vi "Write_SIDto_global_ini.vi"(8 "Error In":errorcluster, 9 "Session id name":string="sid", 10 "SID":string, 11 "Global ini path":path) -> (0 "Error Out":errorcluster)   [LabVIEW 2017]
doc: "This VI records the SID at runtime and place it in Global ini file\n\n\\..\\UltraSonic_Test_Scripts\\UltraSonic_Global_Config.ini"
uses:
  <vilib>/Utility/config.llb/Write Key (String).vi
  <vilib>/Utility/config.llb/NI_LVConfig.lvlib
panel:
  out "found?":bool
  # "WRITE SID TO GLOBAL INI FILE"
  # "ERROR"
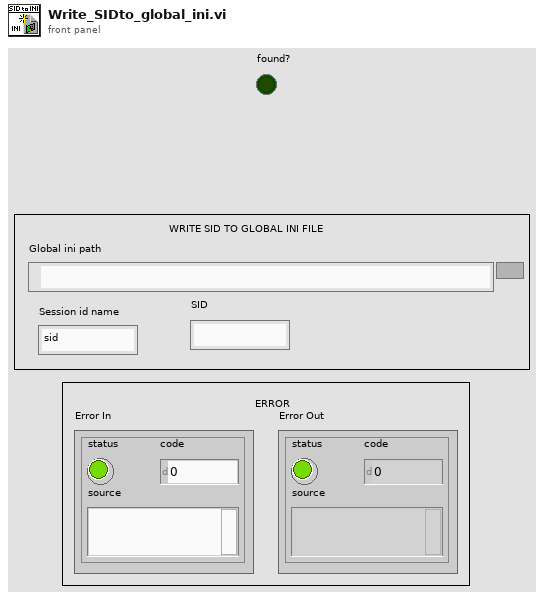
[diagram p1: front panel]
types:
  T1 = typedef "NI_LVConfig.lvlib/Config Data RefNum.ctl" = refnum<k1>
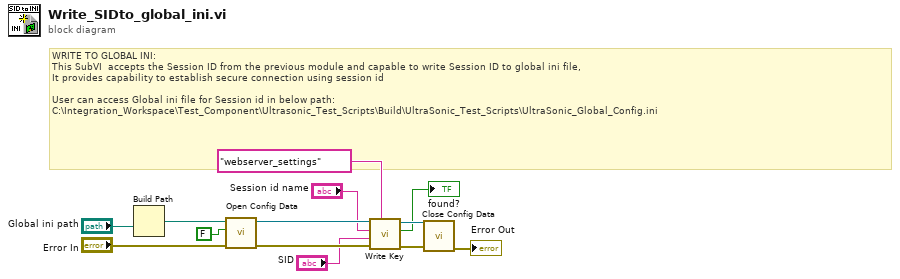
[diagram p0: block diagram]
diagram:
  # "WRITE TO GLOBAL INI:\nThis SubVI  accepts the Session ID from the previous module and capable to write Session ID to global ini file, \nIt provides capability to establish secure connection using session id\n\nUser can access Global ini file for Session id in below path:\nC:\\Integration_Workspace\\Test_Component\\Ultrasonic_Test_Scripts\\Build\\UltraSonic_Test_Scripts\\UltraSonic_Global_Config.ini"
  n1 = Build Path(name or relative path="Global ini path") -> (appended path=w12:path)  [unwired: 1 in]
  n2 = call <vilib>:"Open Config Data.vi"("error in (no error)"="Error In", "create file if necessary (T)"=FALSE ("create file if necessary? (T)"), "configuration file path"=w12) -> ("error out"=w8:errorcluster, "refnum"=w9:T1)  [unwired: 6 in, 1 out]
  n3 = call-poly <vilib>:"Write Key.vi"("section"="webserver_settings", "error in (no error)"=w8, "value"="SID", "key"="Session id name", "refnum"=w9) -> ("error out"=w4:errorcluster, "found?"=→"found?":bool, "refnum out"=w5:T1)  [unwired: 4 in]
  n4 = call <vilib>:"Close Config Data.vi"("error in (no error)"=w4, "refnum"=w5) -> ("error out"=→"Error Out":errorcluster)  [unwired: 8 in, 1 out]
